vi "RecipeFile_Read.vi"(8 "error in (no error)":errorcluster, 11 "file path (dialog if empty)":path) -> (0 "error out":errorcluster)   [LabVIEW 2014]
uses:
  <vilib>/Utility/file.llb/Read From Spreadsheet File (string).vi
panel:
  out "array w/ subset deleted":string[][](array[string])
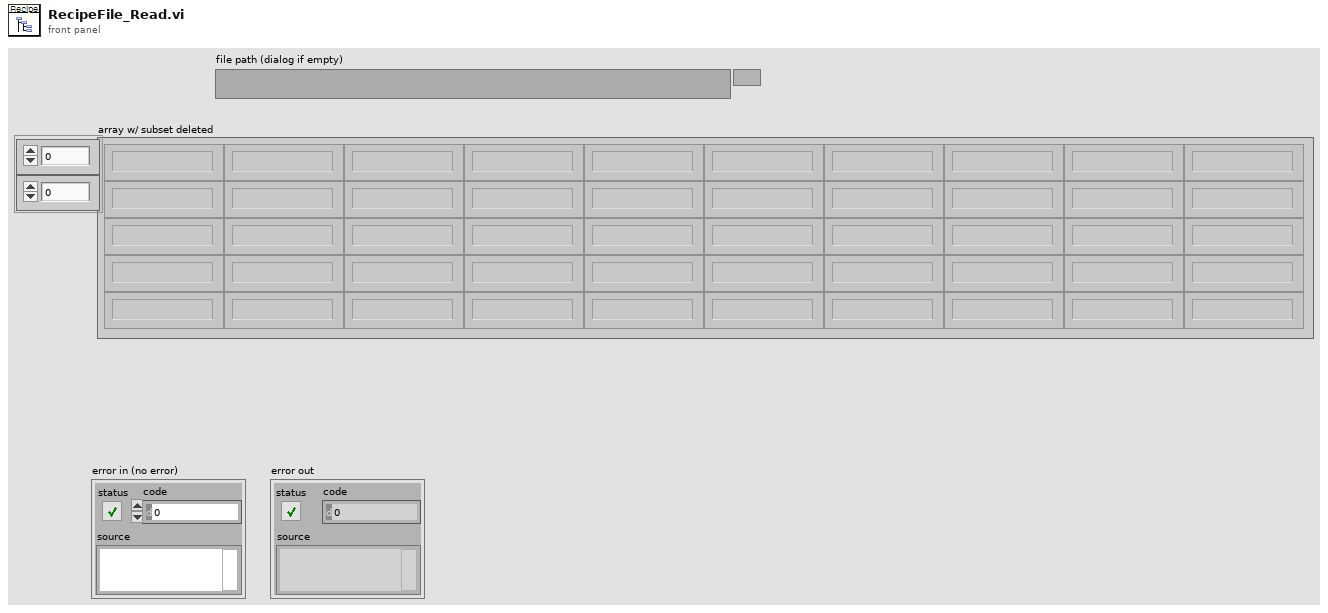
[diagram p1: front panel]
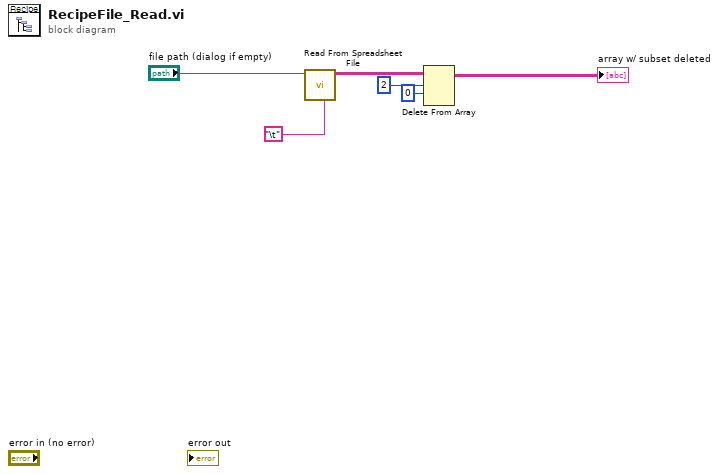
[diagram p0: block diagram]
diagram:
  n1 = call-poly <vilib>:"Read From Spreadsheet File.vi"("delimiter (\\t)"="\t", "file path (dialog if empty)"="file path (dialog if empty)") -> ("all rows"=w4:string[][])  [unwired: 5 in, 4 out]
  n2 = Delete From Array(array=w4, length=2, index (row)=0) -> (array with subset deleted=→"array w/ subset deleted":string[][])  [unwired: 1 in, 1 out]
